vi "GPS.vi"() -> ()   [LabVIEW 2020]
panel:
  out "Fecha":string
  out "Time":string
  out "Ubication":string
  out "A or V":string
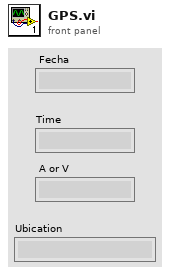
[diagram p1: front panel]
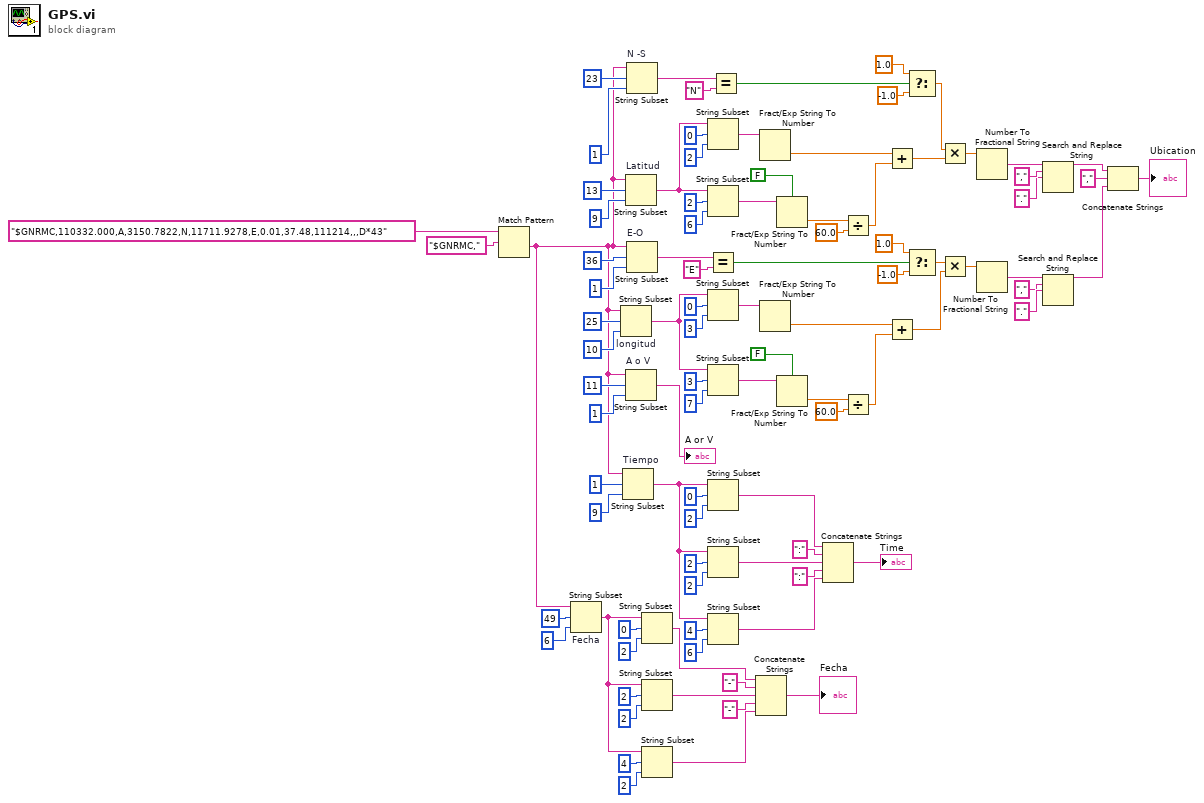
[diagram p0: block diagram]
diagram:
  n1 = Match Pattern(string="$GNRMC,110332.000,A,3150.7822,N,11711.9278,E,0.01,37.48,111214,,,D*43", regular expression="$GNRMC,") -> (after substring=w16:string)  [unwired: 1 in, 3 out]
  n2 = String Subset "Fecha"(string=w16, offset (0)=49, length (rest)=6 ("length (rest)")) -> (substring=w3:string)
  n3 = String Subset "longitud"(string=w16, offset (0)=25, length (rest)=10 ("length (rest)")) -> (substring=w55:string)
  n4 = String Subset "Tiempo"(string=w16, offset (0)=1, length (rest)=9 ("length (rest)")) -> (substring=w26:string)
  n5 = String Subset "Latitud"(string=w16, offset (0)=13, length (rest)=9 ("length (rest)")) -> (substring=w83:string)
  n6 = String Subset "A o V"(string=w16, offset (0)=11, length (rest)=1 ("length (rest)")) -> (substring=→"A or V":string)
  n7 = String Subset "N -S"(string=w16, offset (0)=23, length (rest)=1 ("length (rest)")) -> (substring=w71:string)
  n8 = String Subset "E-O"(string=w16, offset (0)=36, length (rest)=1 ("length (rest)")) -> (substring=w45:string)
  n9 = String Subset(string=w3, offset (0)=0, length (rest)=2 ("length (rest)")) -> (substring=w13:string)
  n10 = String Subset(string=w3, offset (0)=2, length (rest)=2 ("length (rest)")) -> (substring=w11:string)
  n11 = String Subset(string=w3, offset (0)=4, length (rest)=2 ("length (rest)")) -> (substring=w10:string)
  n12 = String Subset(string=w83, offset (0)=0, length (rest)=2 ("length (rest)")) -> (substring=w79:string)
  n13 = String Subset(string=w83, offset (0)=2, length (rest)=6 ("length (rest)")) -> (substring=w80:string)
  n14 = Equal?(x=w45, y="E") -> (x = y?=w47:bool)
  n15 = String Subset(string=w55, offset (0)=0, length (rest)=3 ("length (rest)")) -> (substring=w59:string)
  n16 = String Subset(string=w55, offset (0)=3, length (rest)=7 ("length (rest)")) -> (substring=w58:string)
  n17 = String Subset(string=w26, offset (0)=0, length (rest)=2 ("length (rest)")) -> (substring=w23:string)
  n18 = String Subset(string=w26, offset (0)=2, length (rest)=2 ("length (rest)")) -> (substring=w21:string)
  n19 = String Subset(string=w26, offset (0)=4, length (rest)=6 ("length (rest)")) -> (substring=w19:string)
  n20 = Equal?(x=w71, y="N") -> (x = y?=w69:bool)
  n21 = Concatenate Strings(w13, "-" ("string"), w11, "-" ("string"), w10) -> (→"Fecha":string)
  n22 = Fract/Exp String To Number(string=w79) -> (number=w75:dbl)  [unwired: 3 in, 1 out]
  n23 = Fract/Exp String To Number(string=w59) -> (number=w63:dbl)  [unwired: 3 in, 1 out]
  n24 = Fract/Exp String To Number(use system decimal point (T)=FALSE, string=w80) -> (number=w77:dbl)  [unwired: 2 in, 1 out]
  n25 = Fract/Exp String To Number(use system decimal point (T)=FALSE, string=w58) -> (number=w61:dbl)  [unwired: 2 in, 1 out]
  n26 = Concatenate Strings(w23, ":" ("string"), w21, ":" ("string"), w19) -> (→"Time":string)
  n27 = Divide(x=w77, y=60.0) -> (x/y=w74:dbl)
  n28 = Divide(x=w61, y=60.0) -> (x/y=w64:dbl)
  n29 = Add(x=w75, y=w74) -> (x+y=w65:dbl)
  n30 = Add(x=w63, y=w64) -> (x+y=w44:dbl)
  n31 = Select(t=1.0, s=w69, f=-1.0) -> (s? t:f=w66:dbl)
  n32 = Select(t=1.0, s=w47, f=-1.0) -> (s? t:f=w50:dbl)
  n33 = Multiply(x=w66, y=w65) -> (x*y=w41:dbl)
  n34 = Multiply(x=w50, y=w44) -> (x*y=w40:dbl)
  n35 = Number To Fractional String(number=w41) -> (F-format string=w39:string)  [unwired: 3 in]
  n36 = Number To Fractional String(number=w40) -> (F-format string=w34:string)  [unwired: 3 in]
  n37 = Search and Replace String(input string=w39, search string=",", replace string="." ("replace string (\"\")")) -> (result string=w31:string)  [unwired: 5 in, 3 out]
  n38 = Search and Replace String(input string=w34, search string=",", replace string="." ("replace string (\"\")")) -> (result string=w33:string)  [unwired: 5 in, 3 out]
  n39 = Concatenate Strings(w31, "," ("string"), w33) -> (→"Ubication":string)
